vi "initialize globals.vi"(7 "Def Set":dbl=50.0 caption="Default Setpoint (C)" format="%.2f") -> ()   [LabVIEW 2016]
doc: "This vi initializes the temp control global variables on startup\n\nPaul K Dixon\nPhysics 350\nCSUSB Physics"
uses:
  temp control/globals/temp control global variables.vi
  globals/C(T) global variables.vi
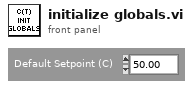
[diagram p1: front panel]
types:
  T1 = typedef "control parameters.ctl" = cluster{"Setpoint":dbl, "Control bandwidth":dbl, "Settle bandwidth":dbl, "Integral time":dbl, "Int\non":bool, "Derivative time":dbl, "Der\non":bool, "Settle time":dbl}
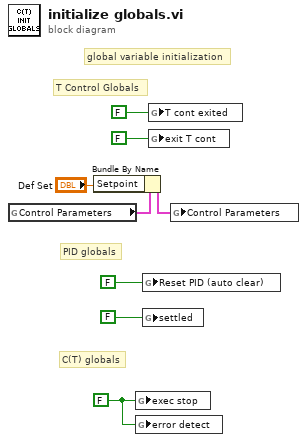
[diagram p0: block diagram]
diagram:
  w4 = FALSE ("exec stop")
  # "C(T) globals"
  # "T Control Globals"
  # "PID globals"
  # "global variable initialization"
  n1 = global read "temp control global variables.vi" "Control Parameters"() -> (w2:T1)
  n2 = Bundle By Name(cluster=w2, "Setpoint"="Def Set") -> (w1:T1)
  n3 = global write "C(T) global variables.vi" "exec stop"(w4) -> ()
  n4 = global write "C(T) global variables.vi" "error detect"(w4) -> ()
  n5 = global write "temp control global variables.vi" "Reset PID (auto clear)"(FALSE ("Reset PID (auto clear)")) -> ()
  n6 = global write "temp control global variables.vi" "settled"(FALSE ("settled")) -> ()
  n7 = global write "temp control global variables.vi" "T cont exited"(FALSE ("T cont exited")) -> ()
  n8 = global write "temp control global variables.vi" "exit T cont"(FALSE ("exit T cont")) -> ()
  n9 = global write "temp control global variables.vi" "Control Parameters"(w1) -> ()
